vi "split object path to hierarchy.vi"(8 "error in (no error)":errorcluster, 11 "Object path":string="IndivITX/Test1/SA03008N.20190801.000000.itx") -> (0 "error out":errorcluster, 1 "layers":i32, 2 "parent path":string, 3 "hierarchy":string[](array[string]))   [LabVIEW 2019, in "LV-Data.S3.lvclass"]
uses:
  LV-Data.S3.lvclass
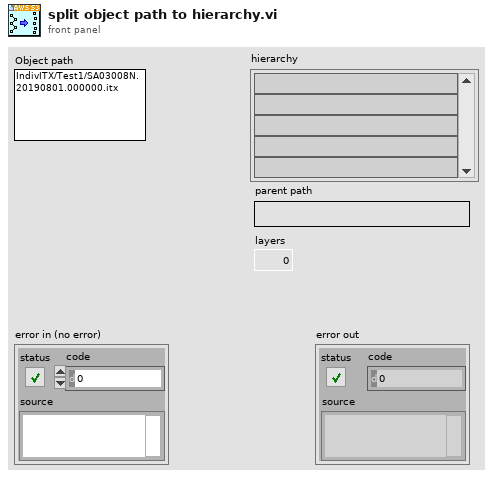
[diagram p1: front panel]
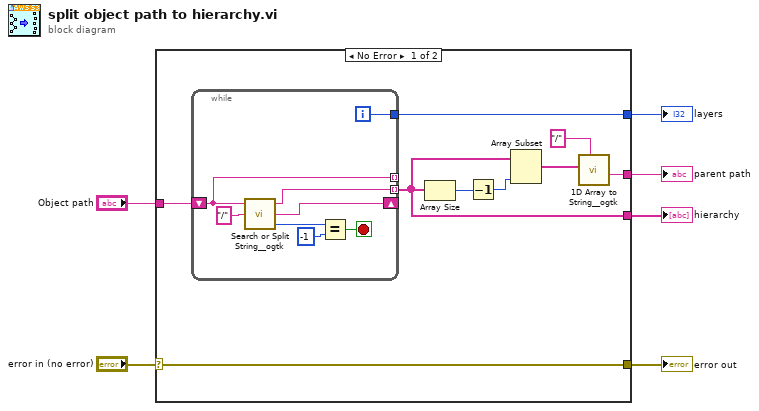
[diagram p0: block diagram]
diagram:
  n1 = case shown="No Error" "error in (no error)" {
    selector: "error in (no error)" -> [w8 w24]
    tunnel: "Object path" -> [w7 _]
    tunnel: [w15 _] -> w5
    tunnel: [w14 _] -> w4
    tunnel: [w10 _] -> w3
    tunnel: [w8 w24] -> w1
    frame No Error {
      n2 = while {
        shift-right: [w16] -> _
        shift-left: w7 -> [w19]
        tunnel: [w19] -> _ mode=indexing
        tunnel: [w18] -> w15
        tunnel: [w17] -> w14 mode=indexing
        i -> [w18]
        stop <- w20 stop-if-true
        n3 = call <userlib>:"Search or Split String__ogtk.vi"("search string/char (-)"="/", "string"=w19) -> ("offset after match"=w22:i32, "substring after match"=w16:string, "substring before match"=w17:string)  [unwired: 1 in]
        n4 = Equal?(x=w22, y=-1) -> (x = y?=w20:bool)
      }
      n5 = Array Size(array=w14) -> (size(s)=w13:i32)
      n6 = Decrement(x=w13) -> (x-1=w12:i32)
      n7 = Array Subset(array=w14, length=w12) -> (w11:string[])  [unwired: 1 in]
      n8 = call <userlib>:"1D Array to String__ogtk.vi"("delimiter (Tab)"="/", "Array of Strings"=w11) -> ("delimited string"=w10:string)  [unwired: 9 in]
    }
    frame Error {
    }
  }
  "hierarchy" <- w4
  "layers" <- w5
  "parent path" <- w3
  "error out" <- w1
